vi "JoystickFunctionL (SubVI).vi"(6 "TimeToReachSpeed":dbl, 7 "DeltaT":dbl, 9 "TweenedSpeed":dbl, 10 "DesiredSpeed":dbl) -> (3 "TweenedJoystick":dbl)   [LabVIEW 2012]
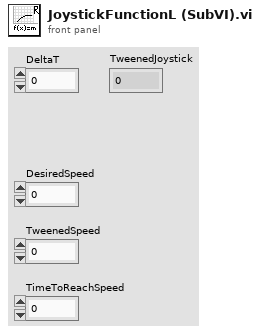
[diagram p1: front panel]
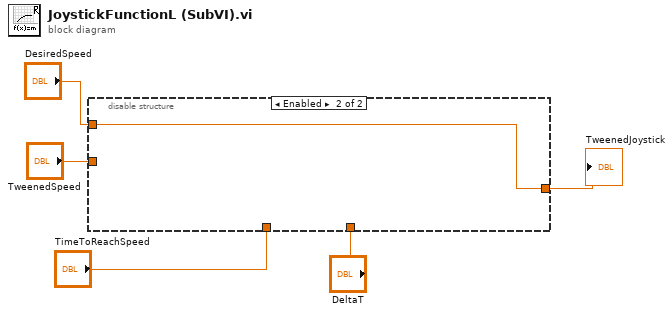
[diagram p0: block diagram]
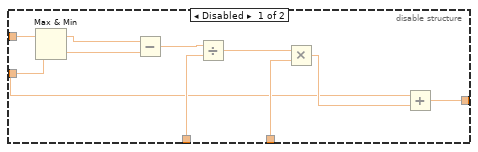
[diagram p2: hidden frame]
diagram:
  n1 = disable-structure shown="Enabled" {
    disable-tunnel: [w15 w16] -> w5
    disable-tunnel: "TimeToReachSpeed" -> [w13 _]
    disable-tunnel: "DeltaT" -> [w12 _]
    disable-tunnel: "DesiredSpeed" -> [w7 w16]
    disable-tunnel: "TweenedSpeed" -> [w6 _]
    frame Disabled {
      n2 = Max & Min(x=w7, y=w6) -> (max(x,y)=w8:dbl, min(x,y)=w9:dbl)
      n3 = Subtract(x=w8, y=w9) -> (x-y=w10:dbl)
      n4 = Divide(x=w10, y=w13) -> (x/y=w11:dbl)
      n5 = Multiply(x=w11, y=w12) -> (x*y=w14:dbl)
      n6 = Add(x=w6, y=w14) -> (x+y=w15:dbl)
    }
    frame Enabled {
    }
  }
  "TweenedJoystick" <- w5
